vi "Read timeouts.vi"(8 "error in (no error)":errorcluster, 11 "MBParam in":refnum<class "TCP Param.lvclass">) -> (0 "error out":errorcluster, 2 "timeouts":T1={"conn_timeout"=1000, "reconn_timeout"=3000, "N attempt max"=3, "t_reset_TTL"=120000, "write_timeout"=50, "read_timeout"=500, "period"=100}, 3 "MBParam out":refnum<class "TCP Param.lvclass">)   [LabVIEW 2021, in "Param.lvlib" / "TCP Param.lvclass"]
uses:
  TCP Param.lvclass
  Typedefs/timeouts.ctl
  TCP Param.lvclass/TCP Param.ctl
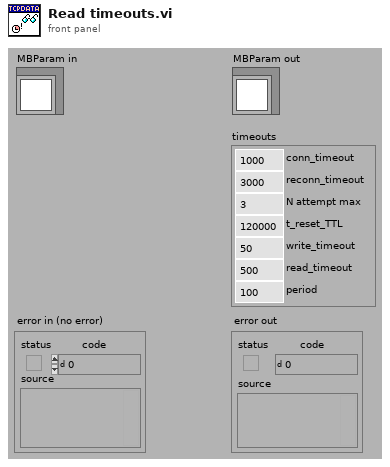
[diagram p1: front panel]
types:
  T1 = typedef "Param.lvlib/TCP Param.lvclass/timeouts.ctl" = cluster{"conn_timeout":i32, "reconn_timeout":i32, "N attempt max":i32, "t_reset_TTL":i32, "write_timeout":i32, "read_timeout":i32, "period":i32}
  T2 = cluster{"IP address":cluster{"Remote IP Address":string, "Remote Port":u16}, "timeouts":T1}
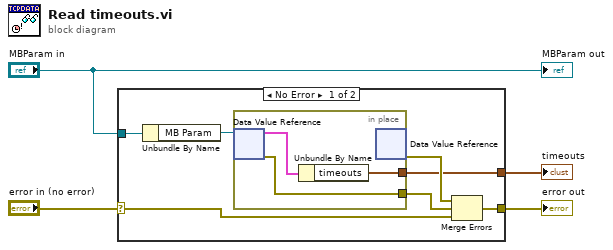
[diagram p0: block diagram]
diagram:
  n1 = case shown="No Error" "error in (no error)" {
    selector: "error in (no error)" -> [w6 w15]
    tunnel: [w10 w15] -> w4
    tunnel: [w5 _] -> w1
    tunnel: "MBParam in" -> [w11 _]
    frame No Error {
      n2 = Unbundle By Name(w11) -> ("MB Param"=w7:refnum<data-value>)
      n3 = in-place {
        in-place-border: [w14] -> w8
        in-place-border: [w12] -> w5
        n4 = in-place-dvr #1(w7) -> (w13:T2, w14:errorcluster)
        n5 = Unbundle By Name(w13) -> ("timeouts"=w12:T1)
        n6 = in-place-dvr #1() -> (w9:errorcluster)  [unwired: 1 in, 1 out]
      }
      n7 = Merge Errors(w9, w8, w6) -> (w10:errorcluster)
    }
    frame Error {
    }
  }
  "error out" <- w4
  "timeouts" <- w1
  "MBParam out" <- "MBParam in"
